vi "Parse_D4.vi"(11 "read buffer":string) -> (2 "D4":bool, 3 "Data":T1 {"Current"."Raw" format="%x"; "Detector"."Raw" format="%x"})   [LabVIEW 2014]
panel:
  out "appended array":string[](array[string])
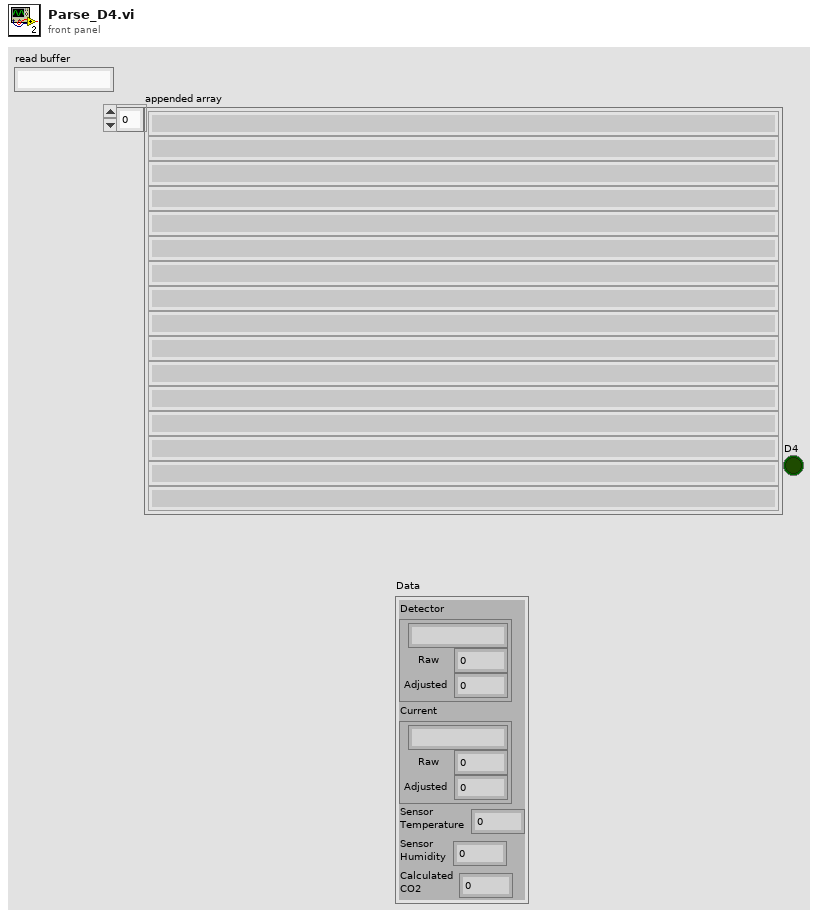
[diagram p1: front panel]
types:
  T1 = cluster{"Detector":cluster{"String":string, "Raw":u16, "Adjusted":dbl}, "Current":cluster{"String":string, "Raw":u16, "Adjusted":dbl}, "Sensor\nTemperature":dbl, "Sensor\nHumidity":dbl, "Calculated\nCO2":dbl}
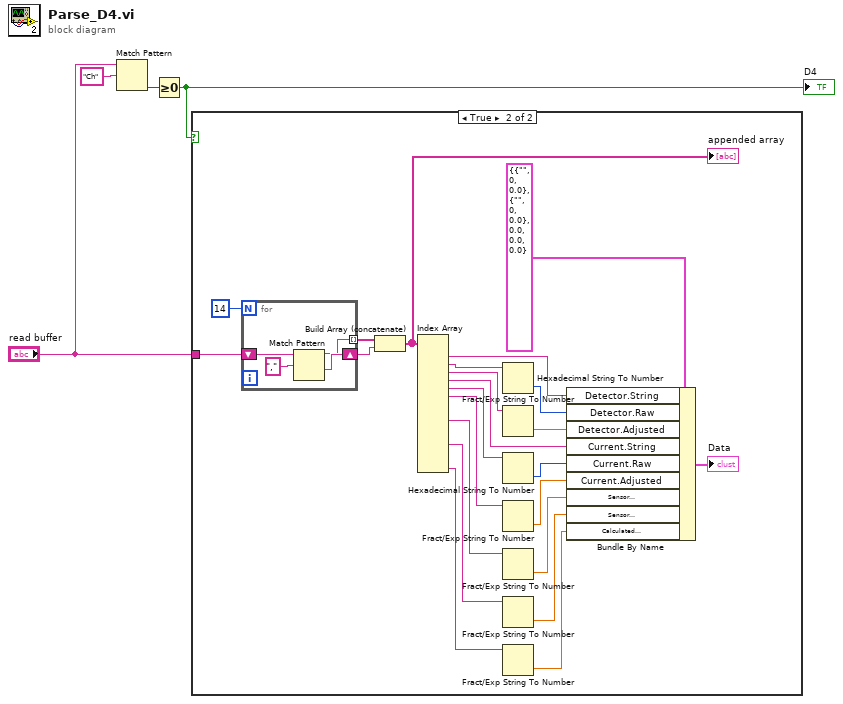
[diagram p0: block diagram]
diagram:
  n1 = Match Pattern(string="read buffer", regular expression="Ch") -> (offset past match=w2:i32)  [unwired: 1 in, 3 out]
  n2 = Greater Or Equal To 0?(x=w2) -> (x >= 0?=w3:bool)
  "D4" <- w3
  n3 = case shown="True" w3 {
    tunnel: "read buffer" -> [_ w27]
    frame False {
    }
    frame True {
      n4 = for {
        N: 14 -> [_]
        shift-right: [w29] -> w24
        shift-left: w27 -> [w31]
        tunnel: [w28] -> w25 mode=indexing
        n5 = Match Pattern(string=w31, regular expression=",") -> (before substring=w28:string, after substring=w29:string)  [unwired: 1 in, 2 out]
      }
      n6 = Build Array (concatenate)(w25, w24) -> (w23:string[])
      "appended array" <- w23
      n7 = Index Array(array=w23) -> (element #1=w13:string, element #2=w22:string, element #3=w21:string, element #4=w10:string, element #5=w20:string, element #6=w19:string, element #9=w18:string, element #12=w17:string, element #15=w16:string)  [unwired: 15 in, 6 out]
      n8 = Hexadecimal String To Number(string=w22) -> (number=w11:u32)  [unwired: 2 in, 1 out]
      n9 = Fract/Exp String To Number(string=w21) -> (number=w12:dbl)  [unwired: 3 in, 1 out]
      n10 = Hexadecimal String To Number(string=w20) -> (number=w9:u32)  [unwired: 2 in, 1 out]
      n11 = Fract/Exp String To Number(string=w19) -> (number=w8:dbl)  [unwired: 3 in, 1 out]
      n12 = Fract/Exp String To Number(string=w18) -> (number=w7:dbl)  [unwired: 3 in, 1 out]
      n13 = Fract/Exp String To Number(string=w17) -> (number=w6:dbl)  [unwired: 3 in, 1 out]
      n14 = Fract/Exp String To Number(string=w16) -> (number=w5:dbl)  [unwired: 3 in, 1 out]
      n15 = Bundle By Name(cluster=T1 {"Detector"={"String"="", "Raw"=0, "Adjusted"=0.0}, "Current"={"String"="", "Raw"=0, "Adjusted"=0.0}, "Sensor\nTemperature"=0.0, "Sensor\nHumidity"=0.0, "Calculated\nCO2"=0.0} ("Data"), "Detector.String"=w13, "Detector.Raw"=w11, "Detector.Adjusted"=w12, "Current.String"=w10, "Current.Raw"=w9, "Current.Adjusted"=w8, "Sensor\nTemperature"=w7, "Sensor\nHumidity"=w6, "Calculated\nCO2"=w5) -> (→"Data":T1)
    }
  }
